vi "Go_to_Idle.vi"(8 "error in (no error)":errorcluster, 10 "Nested in":refnum<class "ATM_UI_Controller.lvclass">, 11 "User_Console in":refnum<class "User_Console.lvclass">) -> (0 "error out":errorcluster, 3 "State out":refnum<class "State Actor.lvclass">)   [LabVIEW 2025, in "User_Console.lvlib" / "User_Console.lvclass"]
uses:
  User_Console.lvclass
  C:/Program Files (x86)/National Instruments/LabVIEW 2025/vi.lib/ActorFramework/Actor/Actor.lvclass
  C:/Program Files (x86)/National Instruments/LabVIEW 2025/vi.lib/ni/Actors/State Actor/State Actor/State Actor.lvclass
  <vilib>/ni/Actors/State Actor/State Actor/State Actor.lvclass
  ATM_UI_Controller/ATM_UI_Controller.lvclass
  UC_Idle/UC_Idle.lvclass
  <vilib>/ActorFramework/Actor/Actor.lvclass/Actor.ctl
  ATM_UI_Controller Messages/Update_Message Msg/Update_Message Msg.lvclass/Update_Message Msg.ctl
  <vilib>/ActorFramework/Message Enqueuer/Message Enqueuer.lvclass/Message Enqueuer.ctl
  ATM_UI_Controller Messages/Update_Current_trans Msg/Update_Current_trans Msg.lvclass/Update_Current_trans Msg.ctl
  <vilib>/ActorFramework/Message Enqueuer/Enqueue.vi
  ATM_UI_Controller Messages/Update_Message Msg/Update_Message Msg.lvclass
  C:/Program Files (x86)/National Instruments/LabVIEW 2025/vi.lib/ActorFramework/Message/Message.lvclass
  ATM_UI_Controller Messages/Update_Current_trans Msg/Update_Current_trans Msg.lvclass
  <vilib>/ActorFramework/Message Priority Queue/Priority Enqueue.vi
  User_Console.lvclass/User_Console.ctl
  <vilib>/ActorFramework/Actor/Actor.lvclass
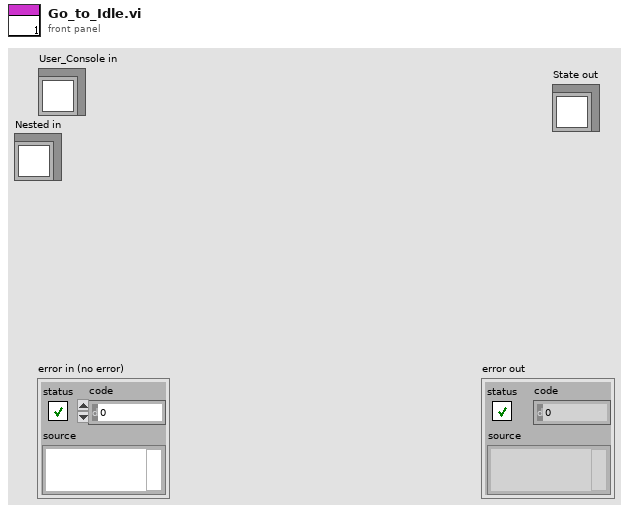
[diagram p1: front panel]
types:
  T1 = cluster{"Message":string, "CARD_READ":bool, "Nested in":refnum<class "ATM_UI_Controller.lvclass">}
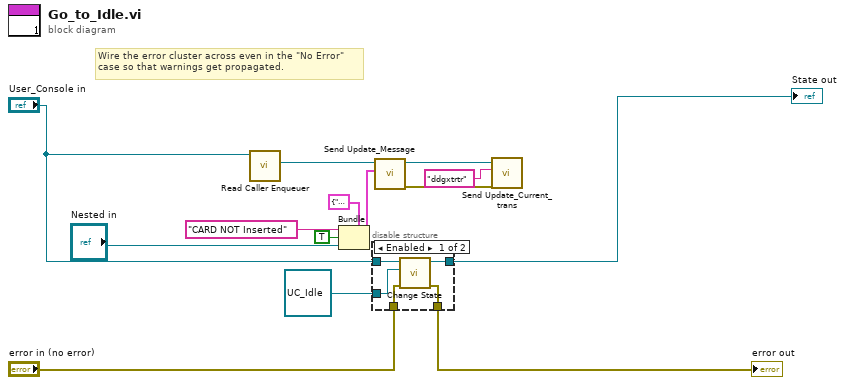
[diagram p0: block diagram]
diagram:
  # "Wire the error cluster across even in the \"No Error\"\ncase so that warnings get propagated."
  n1 = call <vilib>:"Read Caller Enqueuer.vi"("Actor"="User_Console in") -> ("Caller Enqueuer"=w14:refnum<class "Message Enqueuer.lvclass">)  [unwired: 10 in]
  n2 = Bundle(cluster=T1 {"Message"="", "CARD_READ"=FALSE, "Nested in"=refnum} ("Message"), "Message"="CARD NOT Inserted", "CARD_READ"=TRUE, "Nested in"="Nested in") -> (w2:T1)
  n3 = disable-structure shown="Enabled" {
    disable-tunnel: refnum<class "UC_Idle.lvclass"> refnum ("User_Console.lvlib:UC_Idle.lvclass") -> [w19 _]
    disable-tunnel: [w18 w20] -> w8
    disable-tunnel: "User_Console in" -> [w17 w20]
    disable-tunnel: "error in (no error)" -> [w16 w21]
    disable-tunnel: [w15 w21] -> w5
    frame Enabled {
      n4 = call <vilib>:"Change State.vi"("error in (no error)"=w16, "New State in"=w19, "State in"=w17) -> ("error out"=w15:errorcluster, "State out"=w18:refnum<class "State Actor.lvclass">)  [unwired: 7 in]
    }
    frame Disabled {
    }
  }
  "error out" <- w5
  "State out" <- w8
  n5 = call "Send Update_Message.vi"("Message"=w2, "Message Enqueuer"=w14) -> ("error out"=w4:errorcluster, "Message Enqueuer out"=w13:refnum<class "Message Enqueuer.lvclass">)  [unwired: 8 in]
  n6 = call "Send Update_Current_trans.vi"("error in (no error)"=w4, "Current Transaction"="ddgxtrtr", "Message Enqueuer"=w13) -> ()  [unwired: 7 in, 2 out]
